vi "h.SENSORS.GetSensorNames.vi"(8 "error in":errorcluster, 11 "Connection ID":refnum<k5>) -> (0 "error out":errorcluster, 2 "Sensor Names":string[](array[string]), 3 "Connection ID out":refnum<k5>)   [LabVIEW 2016, in "h.Library.lvlib"]
uses:
  h.Library.lvlib
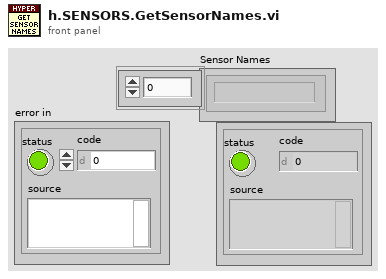
[diagram p1: front panel]
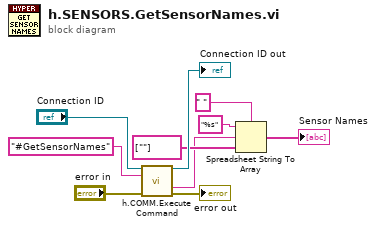
[diagram p0: block diagram]
diagram:
  n1 = call "h.COMM.Execute Command.vi"("Connection ID"="Connection ID", "Command"="#GetSensorNames", "error in"="error in") -> ("Connection ID out"=→"Connection ID out":refnum<k5>, "Message"=w2:string, "error out"=→"error out":errorcluster)  [unwired: 5 in, 5 out]
  n2 = Spreadsheet String To Array(delimiter (Tab)=" ", format string="%s", spreadsheet string=w2, array type (2D Dbl)=string[] [""]) -> (array=→"Sensor Names":string[])
